vi "BuildFilePath.vi"(11 "File Paths":T1={"Local Save Path"=path "\\\\smbhome.uscs.susx.ac.uk\\cv222/Desktop/data", "Newton Save Path"=path "Z:/#Projects/Entanglement/data", "File Name"="test", "LocalSave"=TRUE}) -> (3 "appended path":path)   [LabVIEW 2019]
uses:
  controls/FilePaths.ctl
  controls/GlobalExp.vi
  Global.lvlib
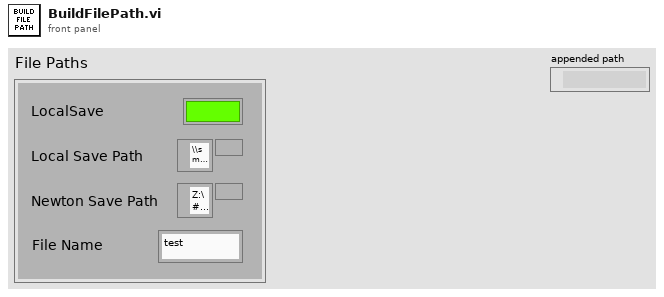
[diagram p1: front panel]
types:
  T1 = typedef "FilePaths.ctl" = cluster{"Local Save Path":path, "Newton Save Path":path, "File Name":string, "LocalSave":bool}
  T2 = typedef "MasterExpControl.ctl" = cluster{"Main Steps":dbl, "Main Runs":dbl, "ExpStatus":enum16{"Innit", "Stop", "Idle", "MainRunning", "AuxRunning"}, "Main Current Step":dbl, "ExpNum":dbl, "NewData":bool, "date":string, "command":string, "Stop":bool, "Pause":bool, "Mathematica":string, "Main/Meta":bool, "UpdateMath":bool, "Camera":bool, "MetaExpOver":bool, "NextMetaExp":bool}
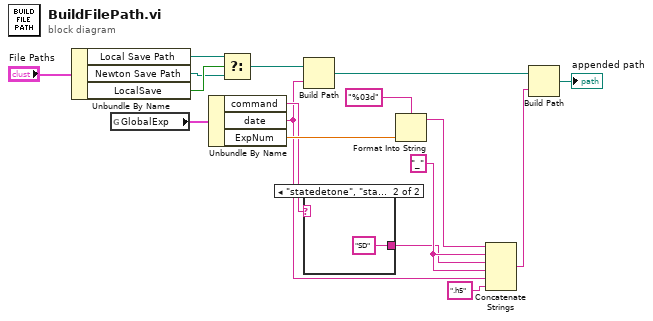
[diagram p0: block diagram]
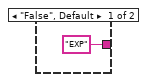
[diagram p2: hidden frame]
diagram:
  w6 = "_"
  n1 = Unbundle By Name("File Paths") -> ("Local Save Path"=w15:path, "Newton Save Path"=w16:path, "LocalSave"=w17:bool)
  n2 = global read "GlobalExp.vi" "GlobalExp"() -> (w9:T2)
  n3 = Unbundle By Name(w9) -> ("command"=w7:string, "date"=w5:string, "ExpNum"=w8:dbl)
  n4 = Select(t=w15, s=w17, f=w16) -> (s? t:f=w12:path)
  n5 = Build Path(base path=w12, name or relative path=w5) -> (appended path=w11:path)
  n6 = case shown="\"statedetone\", \"statedettwo\"" w7 {
    tunnel: ["EXP" "SD"] -> w2
    frame "False", Default {
    }
    frame "statedetone", "statedettwo" {
    }
  }
  n7 = Format Into String(format string="%03d", w8) -> (resulting string=w3:string)  [unwired: 2 in, 1 out]
  n8 = Concatenate Strings(w3, w6, w2, w6, w5, ".h5") -> (w14:string)
  n9 = Build Path(base path=w11, name or relative path=w14) -> (appended path=→"appended path":path)
